vi "onGetVarietal.vi"(8 "error in (no error)":errorcluster, 11 "Leaf in":refnum<class "Leaf.lvclass">) -> (0 "error out":errorcluster, 2 "Varietal":string, 3 "Leaf out":refnum<class "Leaf.lvclass">)   [LabVIEW 2021, in "Bananas.lvlib" / "Leaf.lvclass"]
uses:
  Leaf.lvclass
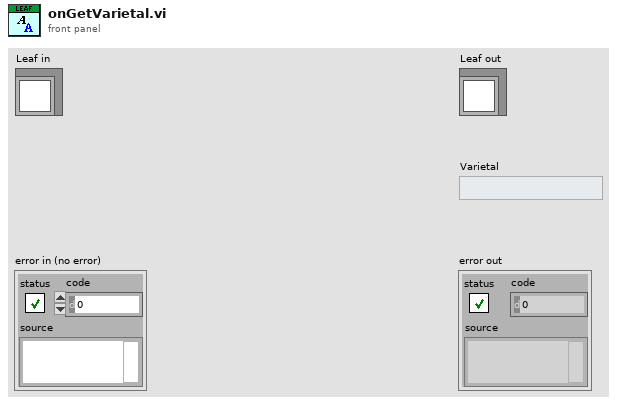
[diagram p1: front panel]
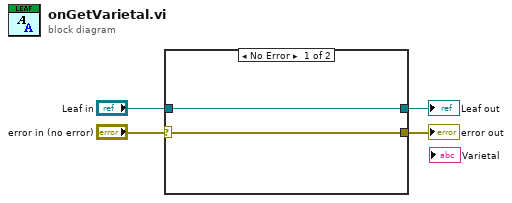
[diagram p0: block diagram]
diagram:
  n1 = case shown="No Error" "error in (no error)" {
    selector: "error in (no error)" -> [w5 w8]
    tunnel: [w5 w8] -> w3
    tunnel: [w6 w7] -> w1
    tunnel: "Leaf in" -> [w6 w7]
    frame No Error {
    }
    frame Error {
    }
  }
  "error out" <- w3
  "Leaf out" <- w1
